vi "Process PAS Waveform Data.vi"() -> ()   [LabVIEW 2014]
panel:
  out "cancelled":bool
  out "Numeric Control":i32
  out "time stamp":timestamp
  out "Waveform Graph 2":i16[][](graph)
  out "Waveform Graph":i16[][](graph)
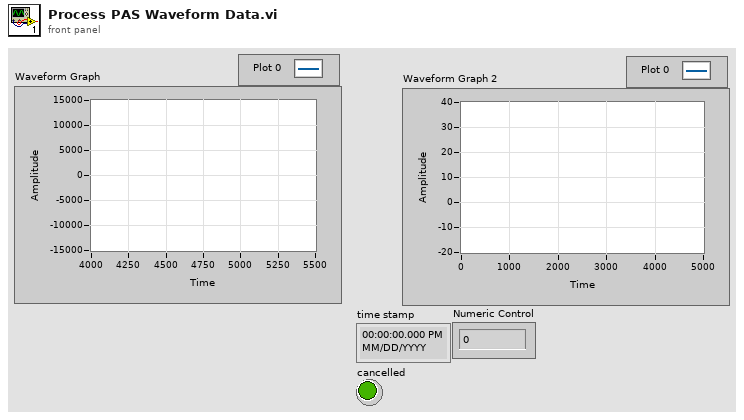
[diagram p1: front panel]
types:
  T1 = enum16{"open", "replace", "create", "open or create", "replace or create", "replace or create with confirmation"}
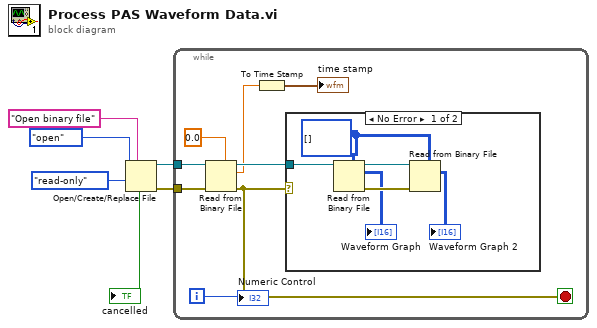
[diagram p0: block diagram]
diagram:
  n1 = Open/Create/Replace File(prompt="Open binary file", operation (0:open)=T1."open", access (0:read/write)=enum16{"read/write", "read-only", "write-only"}."read-only") -> (refnum out=w6:refnum<file>, cancelled=→"cancelled":bool, error out=w5:errorcluster)  [unwired: 3 in]
  n2 = while {
    tunnel: w6 -> [w11]
    tunnel: w5 -> [w10]
    i -> [w7]
    stop <- w14 stop-if-true
    n3 = Read from Binary File(5:0.0, 8:w10, 11:w11) -> (0:w14:errorcluster, 2:w9:dbl, 3:w13:refnum<file>)  [unwired: 3 in, 1 out]
    n4 = To Time Stamp(1:w9) -> (0:→"time stamp":timestamp)
    n5 = case shown="No Error" w14 {
      tunnel: w13 -> [w20 _]
      frame No Error {
        w17 = i16[][] []
        n6 = Read from Binary File(5:w17, 11:w20) -> (0:w18:errorcluster, 2:→"Waveform Graph":i16[][], 3:w19:refnum<file>)  [unwired: 4 in, 1 out]
        n7 = Read from Binary File(5:w17, 8:w18, 11:w19) -> (2:→"Waveform Graph 2":i16[][])  [unwired: 3 in, 3 out]
      }
      frame Error {
      }
    }
    "Numeric Control" <- w7
  }
